vi "temp limits.vi.vi"(7 "Temp limits":cluster{"Min (0)":dbl, "Max (25)":dbl}={"Min (0)"=0.0, "Max (25)"=25.0}, 8 "error in (no error)":errorcluster, 10 "TEMP":dbl) -> (0 "error out":errorcluster, 2 "Warning":bool, 3 "Warning Text":string)   [LabVIEW 2014]
doc: "SubVI porównuje temperaturę\nprocesową z zadanymi wartościami granicznymi"
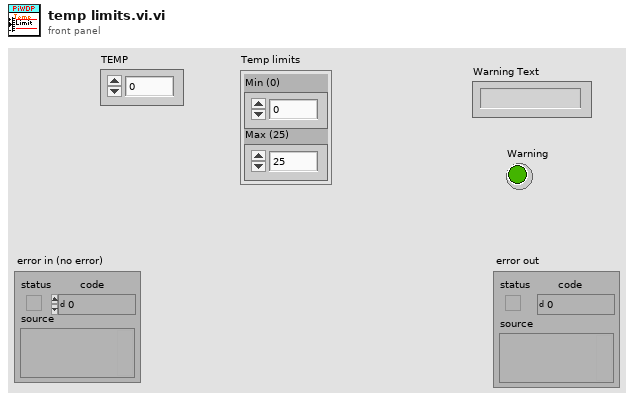
[diagram p1: front panel]
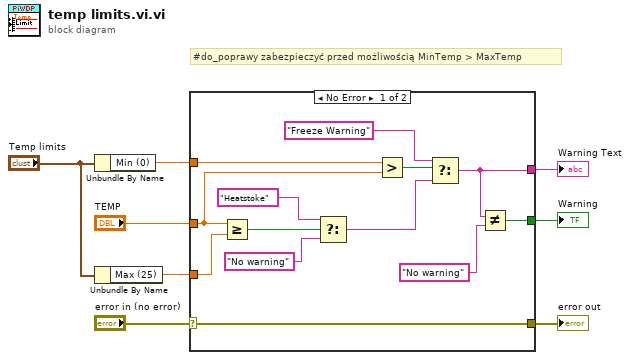
[diagram p0: block diagram]
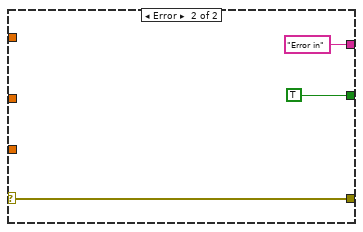
[diagram p2: hidden frame]
diagram:
  # "#do_poprawy zabezpieczyć przed możliwością MinTemp > MaxTemp"
  n1 = Unbundle By Name("Temp limits") -> ("Min (0)"=w3:dbl)
  n2 = Unbundle By Name("Temp limits") -> ("Max (25)"=w2:dbl)
  n3 = case shown="No Error" "error in (no error)" {
    selector: "error in (no error)" -> [w9 w24]
    tunnel: [w9 w24] -> w7
    tunnel: "TEMP" -> [w17 _]
    tunnel: w3 -> [w16 _]
    tunnel: w2 -> [w21 _]
    tunnel: [w12 "Error in"] -> w5
    tunnel: [w10 TRUE] -> w4
    frame No Error {
      n4 = Greater Or Equal?(x=w17, y=w21) -> (x >= y?=w20:bool)
      n5 = Select(t="Heatstoke", s=w20, f="No warning") -> (s? t:f=w14:string)
      n6 = Greater?(x=w16, y=w17) -> (0:w15:bool)
      n7 = Select(t="Freeze Warning", s=w15, f=w14) -> (s? t:f=w12:string)
      n8 = Not Equal?(x=w12, y="No warning") -> (x != y?=w10:bool)
    }
    frame Error {
    }
  }
  "error out" <- w7
  "Warning Text" <- w5
  "Warning" <- w4
